vi "SinusoidalJSMod.vi"(5 "Joystick Input":dbl) -> (2 "Motor Output":dbl)   [LabVIEW 2014]
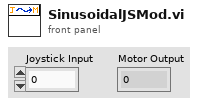
[diagram p1: front panel]
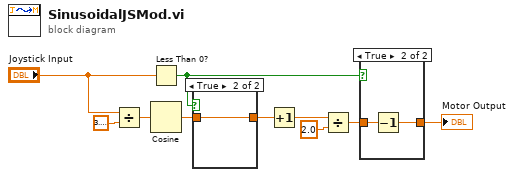
[diagram p0: block diagram]
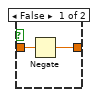
[diagram p3: hidden frame]
diagram:
  n1 = Divide(x="Joystick Input", y=3.141592653589793) -> (x/y=w2:dbl)
  n2 = Less Than 0?(x="Joystick Input") -> (x < 0?=w9:bool)
  n3 = Cosine(x=w2) -> (cos(x)=w6:dbl)
  n4 = case shown="True" w9 {
    tunnel: w6 -> [w12 w13]
    tunnel: [w11 w13] -> w7
    frame False {
      n5 = Negate(x=w12) -> (-x=w11:dbl)
    }
    frame True {
    }
  }
  n6 = Increment(x=w7) -> (x+1=w4:dbl)
  n7 = Divide(x=w4, y=2.0) -> (x/y=w8:dbl)
  n8 = case shown="True" w9 {
    tunnel: w8 -> [w14 w15]
    tunnel: [w14 w16] -> w10
    frame False {
    }
    frame True {
      n9 = Decrement(x=w15) -> (x-1=w16:dbl)
    }
  }
  "Motor Output" <- w10
